vi "execute_value_write_policy.vi"(8 "error in (no error)":errorcluster, 9 "Publish Time":timestamp, 10 "New Topic Value":variant, 11 "TimedAverageSubscription In":refnum<class "TimedAverageSubscription.lvclass">) -> (0 "error out":errorcluster, 3 "TimedAverageSubscription Out":refnum<class "TimedAverageSubscription.lvclass">)   [LabVIEW 2017, in "SubscriptionPolicy.lvlib" / "TimedAverageSubscription.lvclass"]
uses:
  TimedAverageSubscription.lvclass
  C:/Git/mva-framework/Framework/IMediator/ISubscriptionPolicy/ISubscriptionPolicy.lvclass
  TimedAverageSubscription.lvclass/TimedAverageSubscription.ctl
  <vilib>/Composed Systems/Timed Average Buffer/TimedAverageBuffer.lvclass/TimedAverageBuffer.ctl
  IMediator/ISubscriptionPolicy/ISubscriptionPolicy.lvclass/ISubscriptionPolicy.ctl
  <vilib>/Utility/High Resolution Relative Seconds.vi
  IMediator/ITransport/ITransport.lvclass
  IMediator/ISubscriptionPolicy/ISubscriptionPolicy.lvclass
  <vilib>/Composed Systems/Timed Average Buffer/TimedAverageBuffer.lvclass
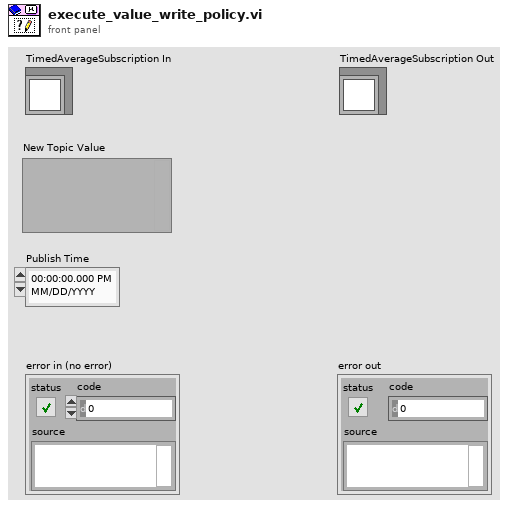
[diagram p1: front panel]
types:
  T1 = typedef "TimedAverageBuffer.lvlib/TimedAverageBuffer.lvclass/TimedAverageBuffer Reference.ctl" = refnum<data-value>
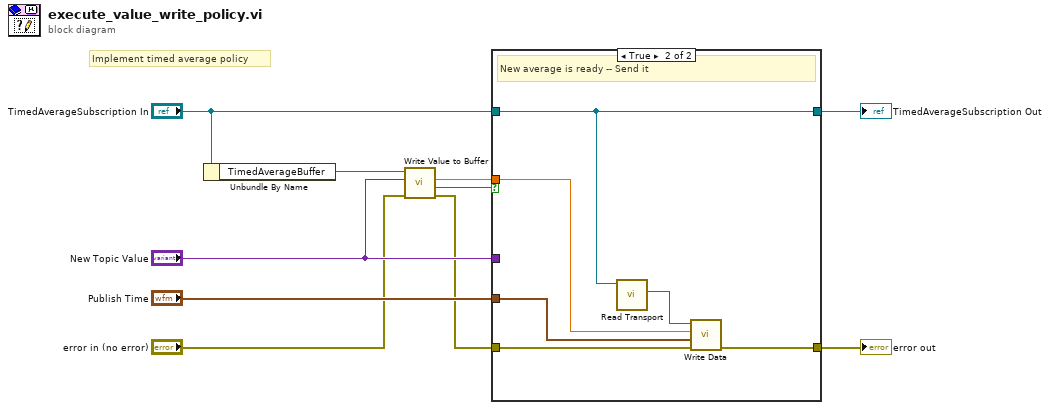
[diagram p0: block diagram]
diagram:
  # "Implement timed average policy"
  n1 = Unbundle By Name("TimedAverageSubscription In") -> ("TimedAverageBuffer"=w6:T1)
  n2 = call <vilib>:"Write Value to Buffer.vi"("error in (no error)"="error in (no error)", "Value"="New Topic Value", "Timed Average Buffer"=w6) -> ("error out"=w1:errorcluster, "New Average Ready?"=w4:bool, "Average"=w3:dbl)  [unwired: 5 in, 1 out]
  n3 = case shown="True" w4 {
    tunnel: "New Topic Value" -> [_ _]
    tunnel: "Publish Time" -> [_ w18]
    tunnel: w1 -> [w11 w14]
    tunnel: [w11 w13] -> w9
    tunnel: "TimedAverageSubscription In" -> [w12 w16]
    tunnel: [w12 w16] -> w7
    tunnel: w3 -> [_ w15]
    frame False {
      # "No new average -- Do nothing"
    }
    frame True {
      # "New average is ready -- Send it"
      n4 = call "Read Transport.vi"("ISubscriptionPolicy in"=w16) -> ("Transport"=w17:refnum<class "ITransport.lvclass">)  [unwired: 10 in]
      n5 = call-dynamic "Write Data.vi"("error in (no error)"=w14, "Publication Time"=w18, "Value"=w15, "ITransport in"=w17) -> ("error out"=w13:errorcluster)  [unwired: 6 in, 1 out]
    }
  }
  "error out" <- w9
  "TimedAverageSubscription Out" <- w7
